vi "make_structure_metaarray.vi"(10 "structure_type":string, 11 "UID":i32) -> (3 "数组":string[](array[string]))   [LabVIEW 2020]
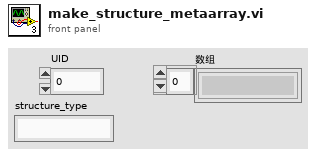
[diagram p1: front panel]
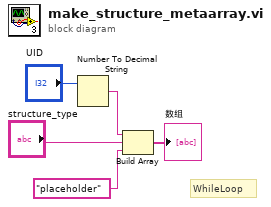
[diagram p0: block diagram]
diagram:
  # "WhileLoop"
  n1 = Number To Decimal String(number="UID") -> (decimal integer string=w3:string)  [unwired: 1 in]
  n2 = Build Array(w3, "structure_type", "placeholder" ("元素")) -> (→"数组":string[])
